vi "U01_9ReadExcelActiveSubVi.vi"() -> ()   [LabVIEW 2019]
panel:
  in  "Multicolumn Listbox":i32(listbox)
  out "data":string[][](array[string])
  out "error out":errorcluster
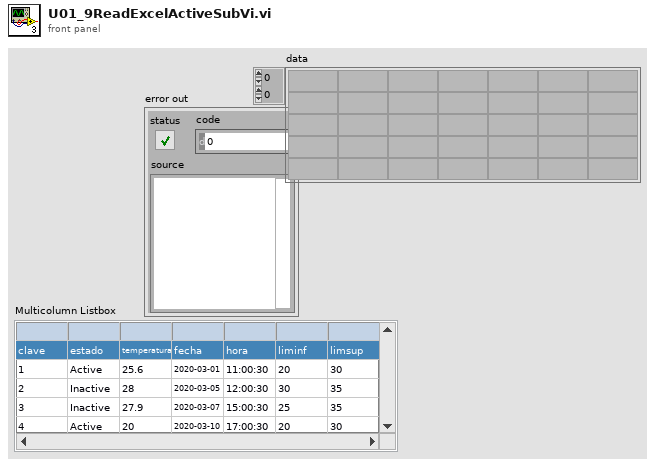
[diagram p1: front panel]
types:
  T1 = cluster{"AppRef":refnum<k7>, "WorkbooksRef":refnum<k7>, "OpenSheetRef":refnum<k7>, "Sheets":refnum<k7>}
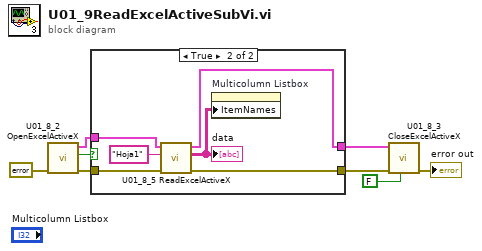
[diagram p0: block diagram]
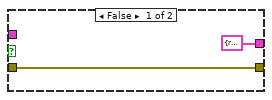
[diagram p2: hidden frame]
diagram:
  n1 = call "U01_8_2 OpenExcelActiveX.vi"("error in"=errorcluster {"status"=FALSE, "code"=0, "source"=""}) -> ("error out"=w6:errorcluster, "IsOpened?"=w1:bool, "Reference"=w8:T1)  [unwired: 8 in]
  n2 = case shown="True" w1 {
    tunnel: w8 -> [_ w16]
    tunnel: [T1 {"AppRef"=refnum, "WorkbooksRef"=refnum, "OpenSheetRef"=refnum, "Sheets"=refnum} ("References") w15] -> w7
    tunnel: w6 -> [w9 w13]
    tunnel: [w9 w12] -> w5
    frame False {
    }
    frame True {
      n3 = call "U01_8_5 ReadExcelActiveX.vi"("error in (no error)"=w13, "NameSheet"="Hoja1", "References"=w16) -> ("error out"=w12:errorcluster, "data"=w11:string[][], "References"=w15:T1)  [unwired: 6 in]
      "data" <- w11
      n4 = property on="Multicolumn Listbox" class="MCListbox (strict)"("ItemNames"=w11) -> ()  [unwired: 2 in, 2 out]
    }
  }
  n5 = call "U01_8_3 CloseExcelActiveX.vi"("Save?"=FALSE, "error in (no error)"=w5, "References"=w7) -> ("error out"=→"error out":errorcluster)  [unwired: 8 in]
